vi "1D Polynomial Evaluation PtByPt.vi"(1 "Coefficients: a":dbl[](array[numeric]), 2 "x":dbl format="%0.2f") -> (0 "y":dbl format="%0.2f")   [LabVIEW 2020, in "NI_PtbyPt.lvlib"]
doc: "Performs a polynomial evaluation of <B>x</B> using <B>Coefficients: a</B>."
uses:
  NI_PtbyPt.lvlib
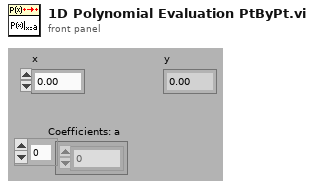
[diagram p1: front panel]
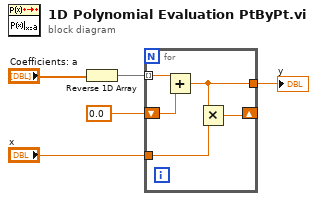
[diagram p0: block diagram]
diagram:
  n1 = Reverse 1D Array(array="Coefficients: a") -> (reversed array=w4:dbl[])
  n2 = for {
    shift-right: [w7] -> _
    shift-left: 0.0 -> [w9]
    tunnel: w4 -> [w10] mode=indexing
    tunnel: "x" -> [w8]
    tunnel: [w6] -> w1
    n3 = Add(x=w10, y=w9) -> (x+y=w6:dbl)
    n4 = Multiply(x=w6, y=w8) -> (x*y=w7:dbl)
  }
  "y" <- w1
